vi "Nickname (Set).vi"(6 "ISOBUS address":T3=-1 caption="ISOBUS address (-1)", 8 "error in":errorcluster, 10 "Nickname":string, 11 "Mercury Reference In":T4) -> (0 "error out":errorcluster, 2 "Response":T1, 3 "Mercury Reference Out":T4, 4 "Valid?":T2)   [LabVIEW 2016, in "Mercury iXX.lvlib" / "Flow.lvlib"]
doc: "Set the Nickname of the selected flow device.\nThe name must be between 1 and 10 alphanumeric characters."
uses:
  Flow.lvlib
  Controls/Mercury Reference.ctl
  Controls/Comms Transport Layer.ctl
  Private/Controls/Query Dynamic Reference.ctl
  Controls/ISOBus Address.ctl
  Controls/Is Valid LED.ctl
  Controls/Response String.ctl
  Private/Controls/Command Verbs.ctl
  Mercury iXX.lvlib
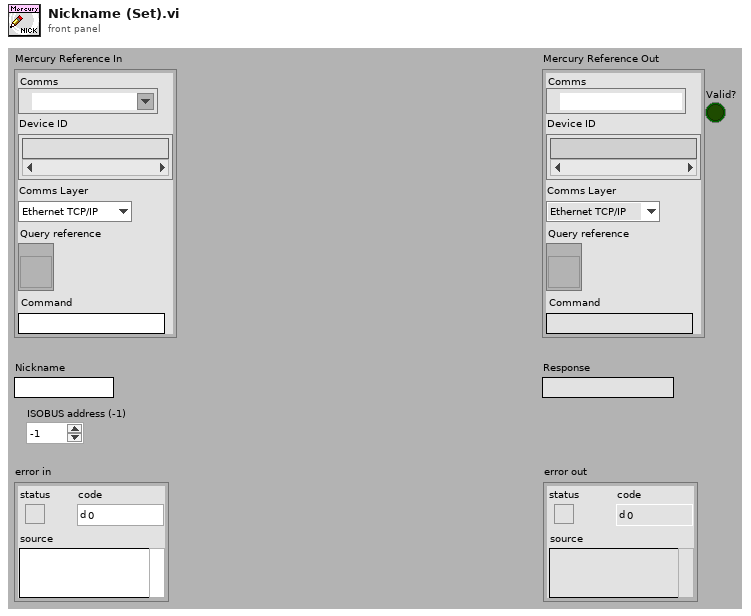
[diagram p1: front panel]
types:
  T1 = typedef "Mercury iXX.lvlib/Response String.ctl" = string
  T2 = typedef "Mercury iXX.lvlib/Is Valid LED.ctl" = bool
  T3 = typedef "Mercury iXX.lvlib/ISOBus Address.ctl" = i32
  T4 = typedef "Mercury iXX.lvlib/Mercury Reference.ctl" = cluster{"Comms":refnum<visa-resource-name>, "Device ID":string[], "Comms Layer":T5, "Command":string, "Query reference":T6}
  T5 = typedef "Mercury iXX.lvlib/Comms Transport Layer.ctl" = enum16{"Ethernet TCP/IP", "USB", "ISOBus - RS-232", "GPIB"}
  T6 = typedef "Mercury iXX.lvlib/Query Dynamic Reference.ctl" = refnum<vi>
  T7 = typedef "Mercury iXX.lvlib/Command Verbs.ctl" = string
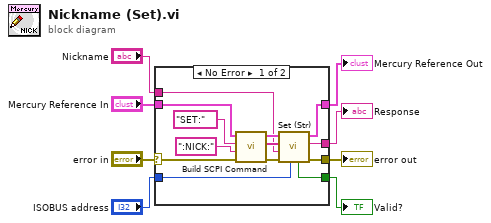
[diagram p0: block diagram]
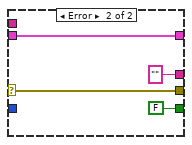
[diagram p2: hidden frame]
diagram:
  n1 = case shown="No Error" "error in" {
    selector: "error in" -> [w9 w25]
    tunnel: [w17 w24] -> w8
    tunnel: [w16 w25] -> w7
    tunnel: [w15 T1 "" ("Response")] -> w6
    tunnel: [w14 T2 FALSE ("Valid?")] -> w5
    tunnel: "ISOBUS address" -> [w13 _]
    tunnel: "Mercury Reference In" -> [w12 w24]
    tunnel: "Nickname" -> [w11 _]
    frame No Error {
      n2 = call "Build SCPI Command.vi"("error in"=w9, "Noun(s)"=":NICK:" ("Command"), "Verb"=T7 "SET:", "Mercury Reference In"=w12) -> ("error out"=w18:errorcluster, "SCPI Message(s)"=w19:string[], "Mercury Reference Out"=w20:T4)  [unwired: 5 out]
      n3 = call "Set (Str).vi"("ISOBUS address"=w13, "error in"=w18, "Command Value (Str)"=w11, "SCPI Message(s)"=w19, "Mercury Reference In"=w20) -> ("error out"=w16:errorcluster, "Response"=w15:T1, "Mercury Reference Out"=w17:T4, "Valid?"=w14:T2)  [unwired: 3 out]
    }
    frame Error {
    }
  }
  "Mercury Reference Out" <- w8
  "error out" <- w7
  "Valid?" <- w5
  "Response" <- w6
